vi "Actor Core.vi"(8 "error in":errorcluster, 11 "Spectroscopy_Controller in":refnum<class "Spectroscopy_Controller.lvclass">) -> (0 "error out":errorcluster, 3 "Actor out":refnum<class "Actor.lvclass">)   [LabVIEW 2023, in "Spectroscopy_Controller.lvlib" / "Spectroscopy_Controller.lvclass"]
doc: "(<B>Filename</B>: Actor Framework.lvlib:Actor.lvclass:Actor Core.vi)\n\nReceives messages to the actor, reacts to them, and initiates any error handling that may shut the actor down.\n\nDescendant classes may override this VI to append parallel tasks for the actor to complete while it handles messages. Overrides use the Call Parent Class Method node."
uses:
  Spectroscopy_Controller.lvclass
  <vilib>/ActorFramework/Actor/Actor.lvclass
  UIs/Camera_Controller/Camera_Controller/Camera_Controller.lvclass
  UIs/SpectrometerUI/SpectrometerUI/SpectrometerUI.lvclass
  <vilib>/ActorFramework/Actor/Actor.lvclass/Actor.ctl
  <vilib>/ActorFramework/Message Enqueuer/Message Enqueuer.lvclass/Message Enqueuer.ctl
  Spectroscopy_Controller.lvclass/Spectroscopy_Controller.ctl
  <vilib>/ActorFramework/Message Enqueuer/Init from Existing Queue.vi
  <vilib>/ActorFramework/Message Enqueuer/Message Enqueuer.lvclass
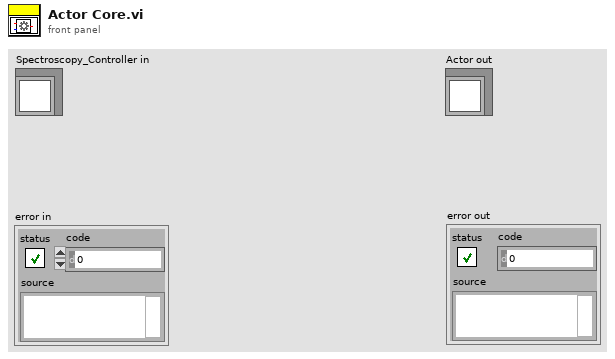
[diagram p1: front panel]
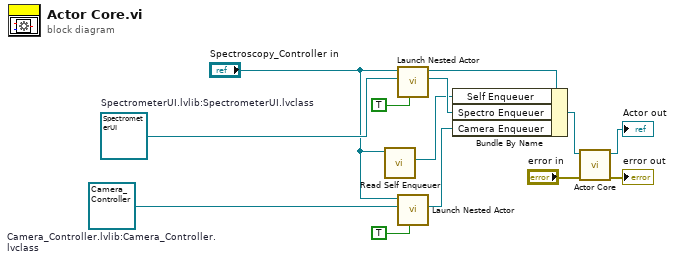
[diagram p0: block diagram]
diagram:
  w4 = refnum<class "SpectrometerUI.lvclass"> refnum  # SpectrometerUI.lvlib:SpectrometerUI.lvclass
  w5 = refnum<class "Camera_Controller.lvclass"> refnum  # Camera_Controller.lvlib:Camera_Controller.lvclass
  n1 = call <vilib>:"Read Self Enqueuer.vi"("Actor"="Spectroscopy_Controller in") -> ("Self Enqueuer"=w1:refnum<class "Message Enqueuer.lvclass">)  [unwired: 10 in]
  n2 = call <vilib>:"Launch Nested Actor.vi"("Open Actor Core front panel? (F)"=TRUE, "Nested Actor"=w4, "Caller Actor in"="Spectroscopy_Controller in") -> ("Nested Actor's Enqueuer"=w6:refnum<class "Message Enqueuer.lvclass">, "Caller Actor out"=w7:refnum<class "Spectroscopy_Controller.lvclass">)  [unwired: 6 in, 1 out]
  n3 = call <vilib>:"Launch Nested Actor.vi"("Open Actor Core front panel? (F)"=TRUE, "Nested Actor"=w5, "Caller Actor in"="Spectroscopy_Controller in") -> ("Nested Actor's Enqueuer"=w8:refnum<class "Message Enqueuer.lvclass">)  [unwired: 6 in, 2 out]
  n4 = Bundle By Name(cluster=w7, "Self Enqueuer"=w1, "Spectro Enqueuer"=w6, "Camera Enqueuer"=w8) -> (w3:refnum<class "Spectroscopy_Controller.lvclass">)
  n5 = call-parent "Actor Core.vi"("error in"="error in", "Actor in"=w3) -> ("error out"=→"error out":errorcluster, "Actor out"=→"Actor out":refnum<class "Actor.lvclass">)  [unwired: 8 in]
